vi "setUp.vi"(8 "error in (no error)":errorcluster, 11 "reference in":refnum<class "Switch Scripting Test Case.lvclass">) -> (0 "error out":errorcluster, 3 "reference out":refnum<class "Switch Scripting Test Case.lvclass">)   [LabVIEW 2017, in "Switch Scripting Test Case.lvclass"]
doc: "setUp runs prior to the test method during test execution. Use this method to initialize any object data required by your tests."
uses:
  Switch Scripting Test Case.lvclass
  C:/Program Files (x86)/National Instruments/LabVIEW 2017/vi.lib/addons/_JKI Toolkits/VI Tester/TestCase.llb/TestCase.lvclass
  NationalInstruments.VeriStand.SystemDefinitionAPI
  Switch Scripting Test Case.lvclass/Switch Scripting Test Case.ctl
  <userlib>/_OpenG.lib/file/file.llb/Append Path to Root if Relative - Scalar__ogtk.vi
  <vilib>/addons/_JKI Toolkits/VI Tester/TestCase.llb/TestCase.lvclass
  niveristand-custom-device-testing-tools/VeriStandTestUtilities/VeriStandTestUtilities.lvlib
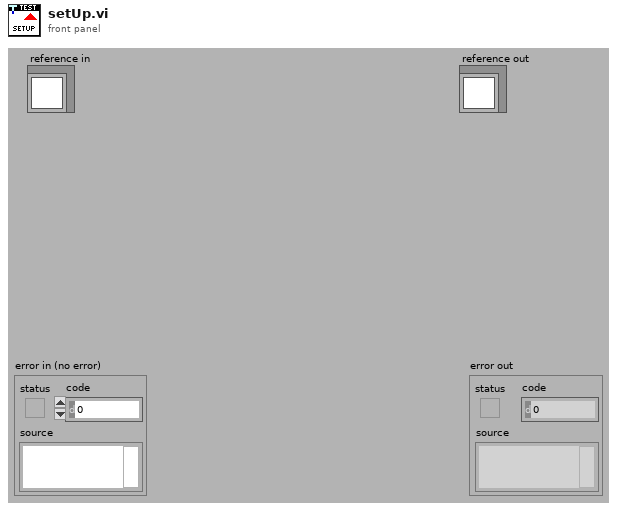
[diagram p1: front panel]
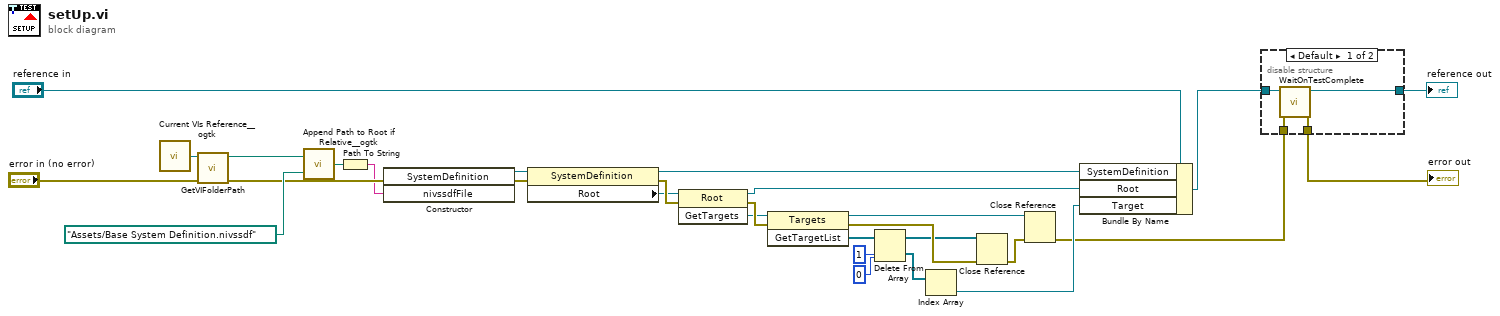
[diagram p0: block diagram]
diagram:
  n1 = call <userlib>:"Current VIs Reference__ogtk.vi"() -> ("Current VI's reference"=w25:refnum<vi>)  [unwired: 5 in]
  n2 = call "GetVIFolderPath.vi"("error in (no error)"="error in (no error)", "VI Reference in"=w25) -> ("error out"=w21:errorcluster, "VI Folder Path out"=w24:path)  [unwired: 8 in]
  n3 = call-poly <userlib>:"Append Path to Root if Relative__ogtk.vi"("Absolute or Relative Path"=path "Assets/Base System Definition.nivssdf", "Root Path"=w24) -> ("Absolute or Appended Path"=w22:path)
  n4 = Path To String(path=w22) -> (string=w19:string)
  n5 = constructor class="SystemDefinition"(error in=w21, "nivssdfFile"=w19) -> (reference out=w18:refnum<k24>, error out=w20:errorcluster)  [unwired: 2 in, 2 out]
  n6 = property class="SystemDefinition"(reference=w18, error in=w20) -> (reference out=w2:refnum<k24>, error out=w17:errorcluster, "Root"=w16:refnum<k24>)
  n7 = invoke class="Root" method="GetTargets"(reference=w16, error in=w17) -> (reference out=w3:refnum<k24>, error out=w15:errorcluster, "GetTargets"=w14:refnum<k24>)  [unwired: 1 in]
  n8 = invoke class="Targets" method="GetTargetList"(reference=w14, error in=w15) -> (reference out=w6:refnum<k24>, error out=w9:errorcluster, "GetTargetList"=w12:refnum<k24>[])  [unwired: 1 in]
  n9 = Delete From Array(array=w12, length=1, index=0) -> (deleted portion=w5:refnum<k24>[], array with subset deleted=w8:refnum<k24>[])
  n10 = Index Array(array=w5) -> (element=w4:refnum<k24>)  [unwired: 1 in]
  n11 = Close Reference(reference=w8, error in (no error)=w9) -> (error out=w7:errorcluster)
  n12 = Close Reference(reference=w6, error in (no error)=w7) -> (error out=w1:errorcluster)
  n13 = Bundle By Name(cluster="reference in", "SystemDefinition"=w2, "Root"=w3, "Target"=w4) -> (w26:refnum<class "Switch Scripting Test Case.lvclass">)
  n14 = disable-structure shown="Default" {
    disable-tunnel: w1 -> [w33 w34]
    disable-tunnel: [w32 w34] -> w29
    disable-tunnel: [w31 w35] -> w27
    disable-tunnel: w26 -> [w30 w35]
    frame condition #0 (active) {
      n15 = call <vilib>:"WaitOnTestComplete.vi"("error in (no error)"=w33, "TestCase in"=w30) -> ("error out"=w32:errorcluster, "TestCase out"=w31:refnum<class "Switch Scripting Test Case.lvclass">)  [unwired: 8 in]
    }
    frame condition #1 {
    }
  }
  "error out" <- w29
  "reference out" <- w27
